vi "function_val.vi"() -> ()   [LabVIEW 2013]
panel:
  out "wynik":dbl
  in  "wartoœæ zadana":dbl
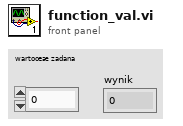
[diagram p1: front panel]
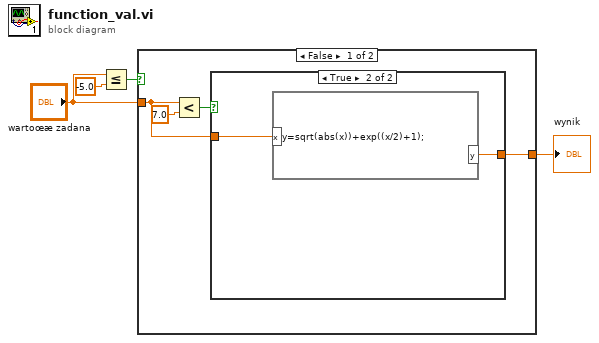
[diagram p0: block diagram]
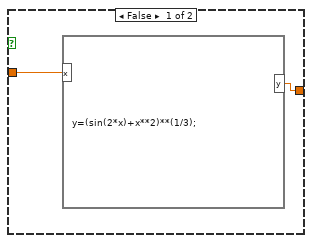
[diagram p2: hidden frame]
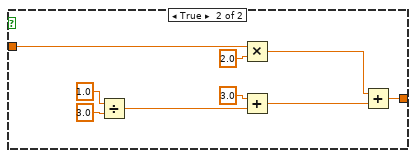
[diagram p3: hidden frame]
diagram:
  n1 = Less Or Equal?(x="wartoœæ zadana", y=-5.0) -> (x <= y?=w4:bool)
  n2 = case shown="False" w4 {
    tunnel: "wartoœæ zadana" -> [w6 w21]
    tunnel: [w5 w13] -> w1
    frame False {
      n3 = Less?(x=w6, y=7.0) -> (x < y?=w8:bool)
      n4 = case shown="True" w8 {
        tunnel: w6 -> [w10 w12]
        tunnel: [w9 w11] -> w5
        frame False {
          n5 = formula code="y=(sin(2*x)+x**2)**(1/3);"("x"=w10) -> ("y"=w9:dbl)
        }
        frame True {
          n6 = formula code="y=sqrt(abs(x))+exp((x/2)+1);"("x"=w12) -> ("y"=w11:dbl)
        }
      }
    }
    frame True {
      n7 = Divide(x=1.0 ("y"), y=3.0) -> (x/y=w14:dbl)
      n8 = Multiply(x=w21, y=2.0) -> (x*y=w19:dbl)
      n9 = Add(x=3.0 ("y"), y=w14) -> (x+y=w17:dbl)
      n10 = Add(x=w19, y=w17) -> (x+y=w13:dbl)
    }
  }
  "wynik" <- w1
